vi "array_intersperse.vi"(2 "Array 2":dbl[](array[numeric]), 3 "Array":dbl[](array[numeric])) -> (0 "Array 3":dbl[](array[numeric]))   [LabVIEW 2015]
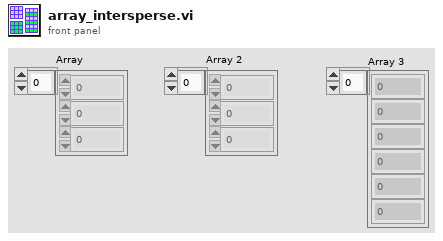
[diagram p1: front panel]
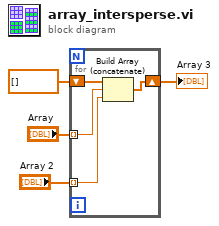
[diagram p0: block diagram]
diagram:
  n1 = for {
    tunnel: "Array" -> [w7] mode=indexing
    tunnel: "Array 2" -> [w6] mode=indexing
    shift-right: [w5] -> w1
    shift-left: dbl[] [] -> [w8]
    n2 = Build Array (concatenate)(w8, w7, w6) -> (w5:dbl[])
  }
  "Array 3" <- w1
